vi "CMD_1.vi"(7 "JsonObj_Ori":refnum<class "JSON Value.lvclass">, 8 "error in (no error)":errorcluster, 9 "F/T":cluster{"Rack":string, "DUT Status":string[]}[](array[cluster])=[{"Rack"="201", "DUT Status"=["READY", "READY", "MAINTAIN", "CLOSE", "TEST"]}, {"Rack"="202", "DUT Status"=["READY", "READY", "MAINTAIN", "READY", "READY"]}], 10 "F/T-B":cluster{"Rack":string, "DUT Status":string[]}[](array[cluster])=[{"Rack"="101", "DUT Status"=["READY", "READY", "MAINTAIN", "CLOSE", "TEST"]}, {"Rack"="102", "DUT Status"=["READY", "READY", "MAINTAIN", "READY", "READY"]}], 11 "H/P":cluster{"Rack":string, "DUT Status":string[]}[](array[cluster])=[{"Rack"="1", "DUT Status"=[]}]) -> (0 "error out":errorcluster, 3 "Result":T1)   [LabVIEW 2020]
uses:
  <vilib>/addons/JSON API/JSON Value/JSON Value.lvclass
  <vilib>/addons/JSON API/JSON Value/Set from JSON string.vi
  <vilib>/addons/JSON API/JSON Value/Set sub-Item by names.vi
  <vilib>/addons/JSON API/JSON Scalar/JSON Scalar.lvclass
  C:/Program Files/National Instruments/LabVIEW 2020/vi.lib/addons/JSON API/JSON Value/JSON Value.lvclass
  <vilib>/addons/JSON API/JSON Array/JSON Array.lvclass
  <vilib>/addons/JSON API/JSON Value/Get sub-Item by names.vi
  <vilib>/addons/JSON API/JSON Scalar/Set String.vi
  <vilib>/addons/JSON API/JSON Value/Set Item by name array.vi
  <vilib>/addons/JSON API/JSON Array/Set JSON Array.vi
  <vilib>/addons/JSON API/JSON Value/Get as JSON string (pretty).vi
  <vilib>/addons/JSON API/Get Polymorphic/JSON GetSet.lvlib
  C:/Program Files/National Instruments/LabVIEW 2020/vi.lib/addons/JSON API/JSON Scalar/JSON Scalar.lvclass
  C:/Program Files/National Instruments/LabVIEW 2020/vi.lib/addons/JSON API/JSON Array/JSON Array.lvclass
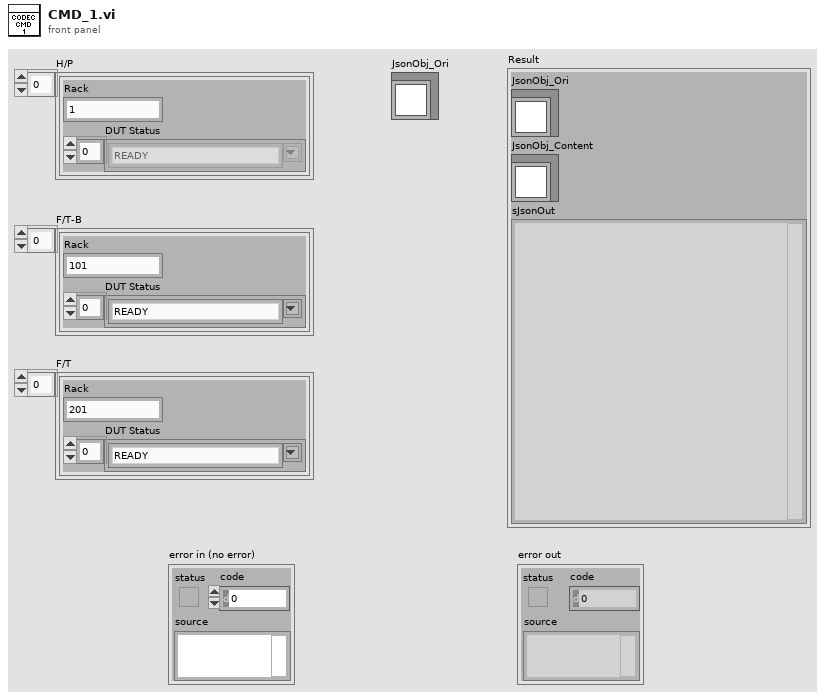
[diagram p1: front panel]
types:
  T1 = cluster{"JsonObj_Ori":refnum<class "JSON Value.lvclass">, "JsonObj_Content":refnum<class "JSON Value.lvclass">, "sJsonOut":string}
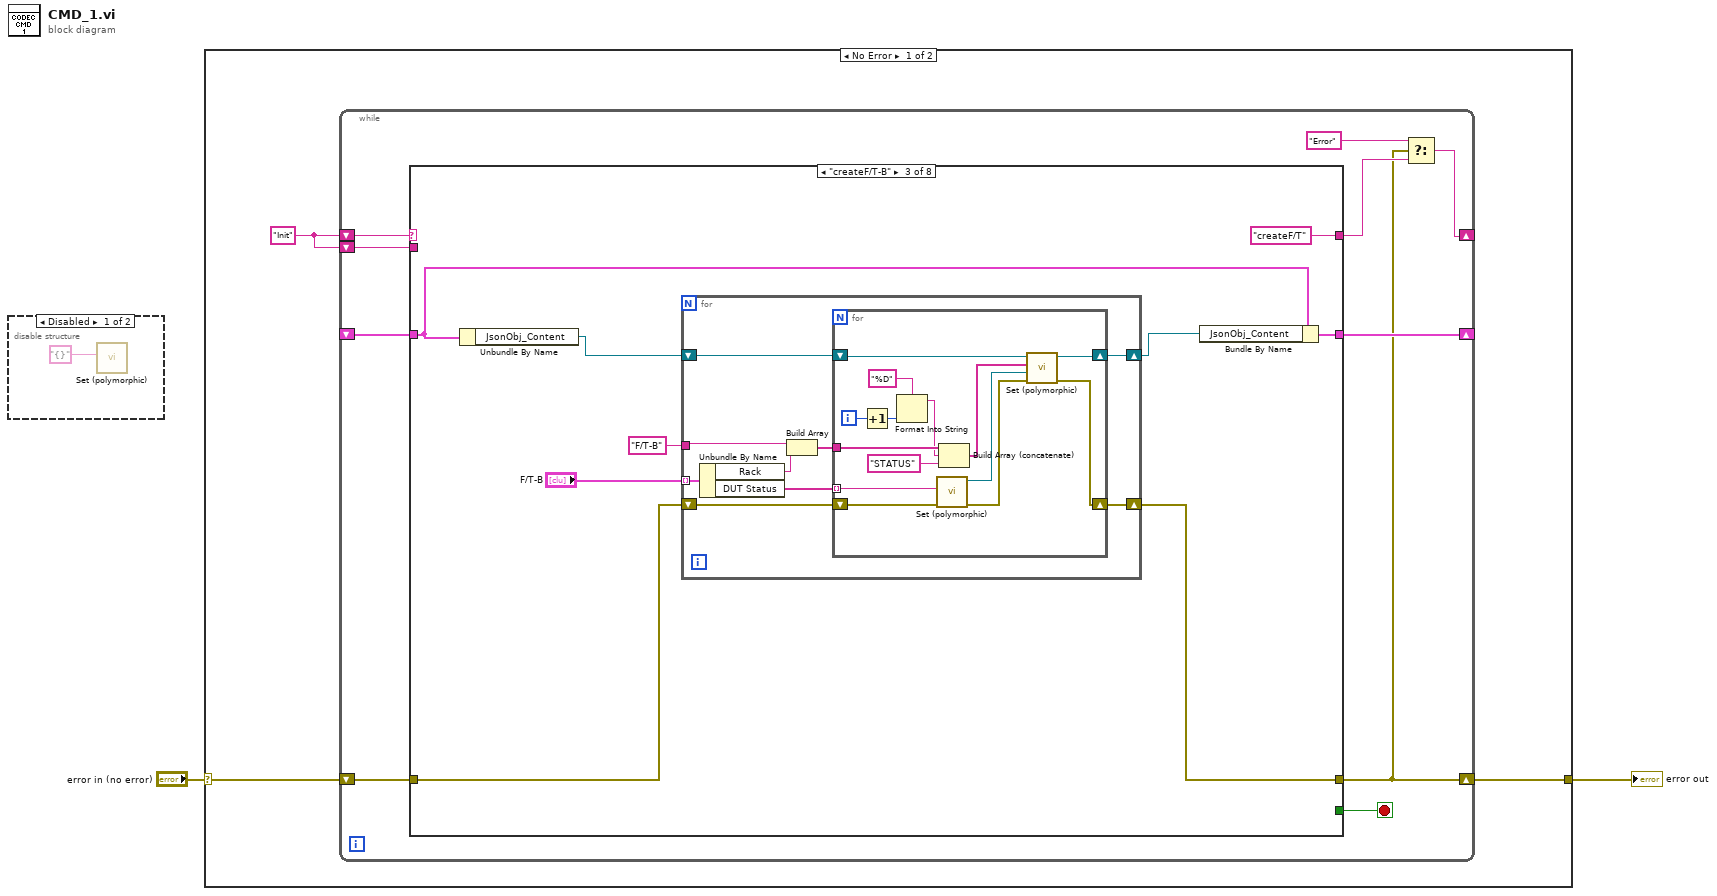
[diagram p0: block diagram]
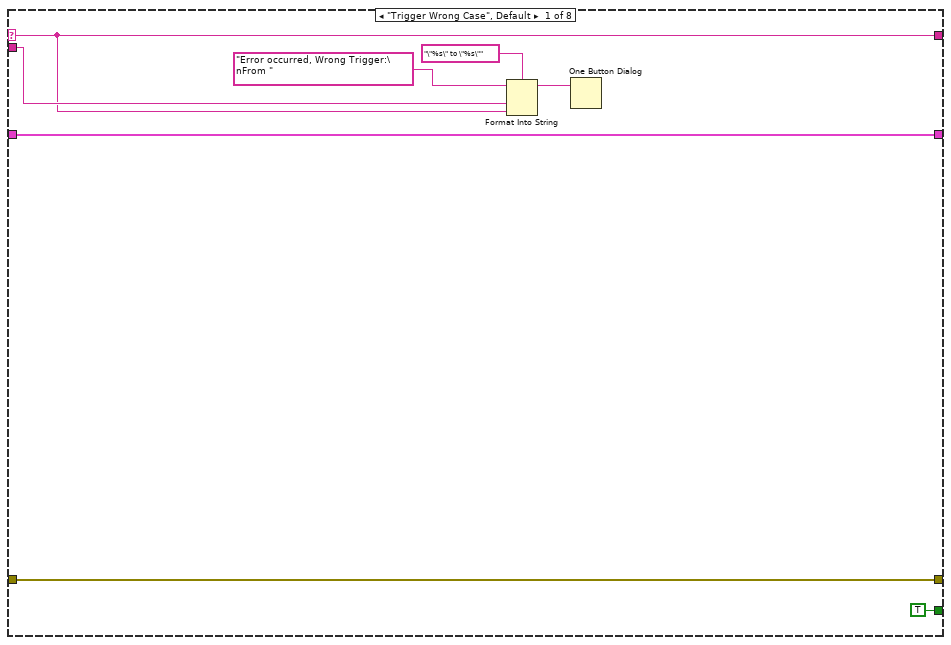
[diagram p3: hidden frame]
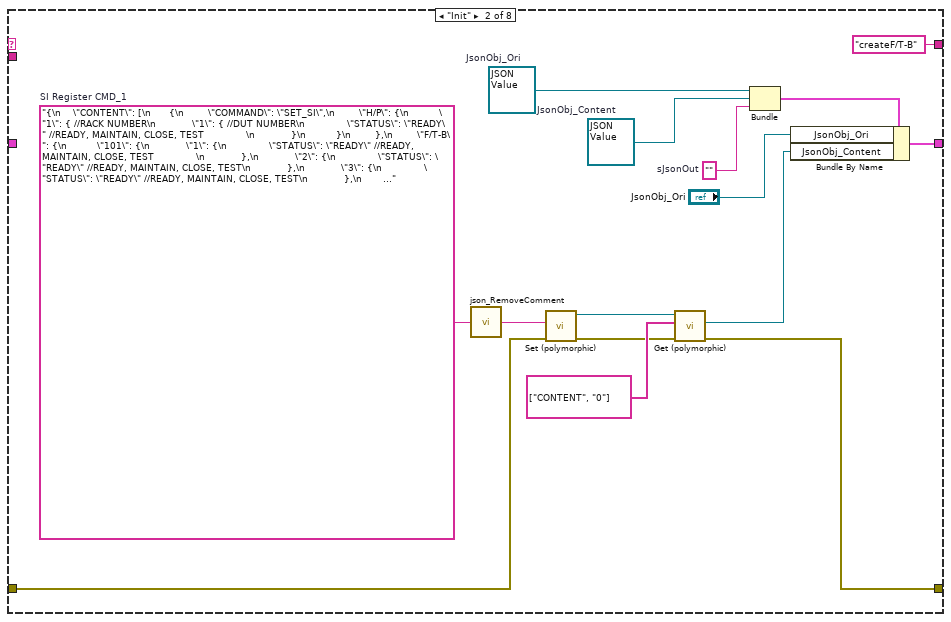
[diagram p4: hidden frame]
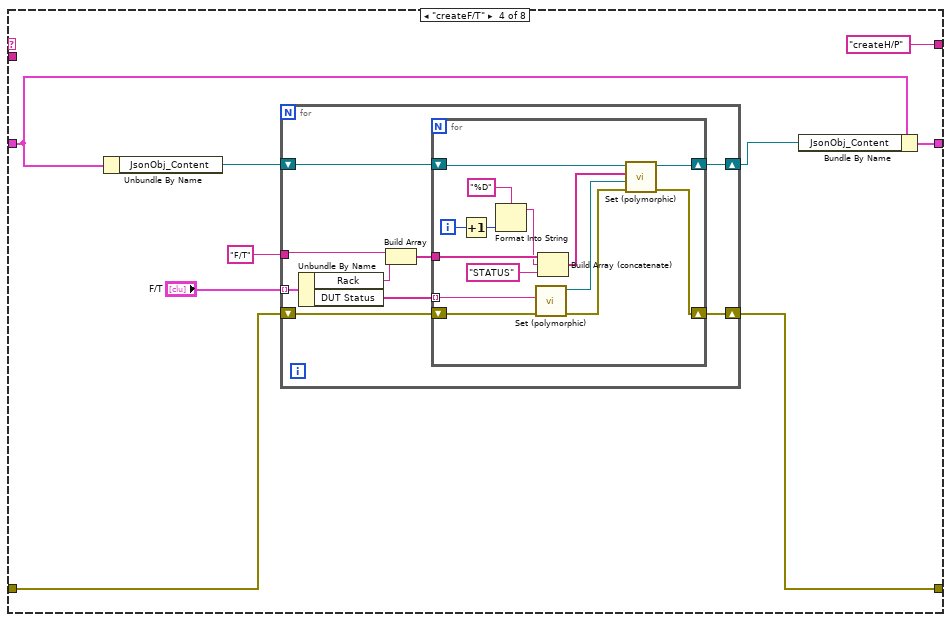
[diagram p5: hidden frame]
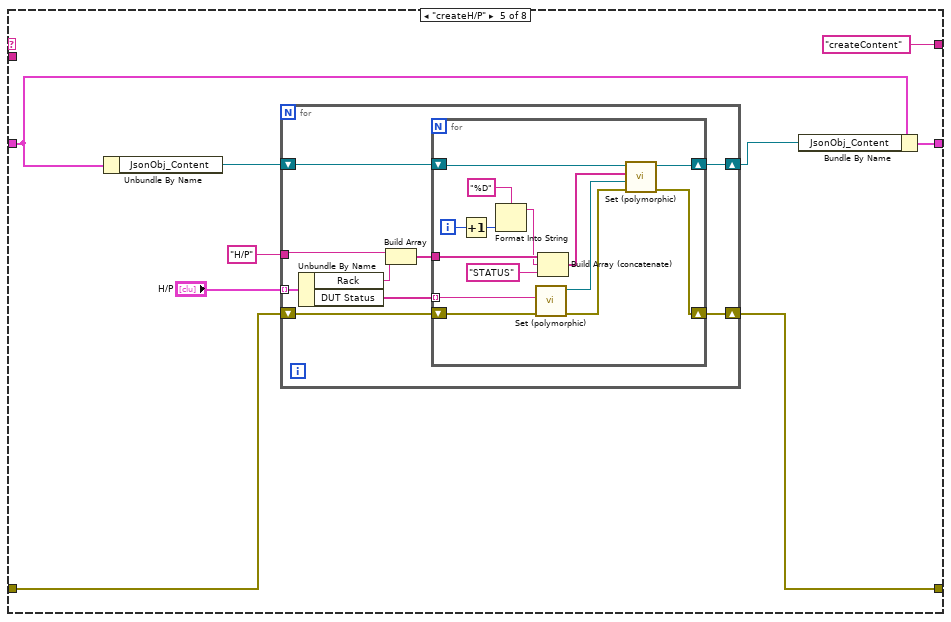
[diagram p6: hidden frame]
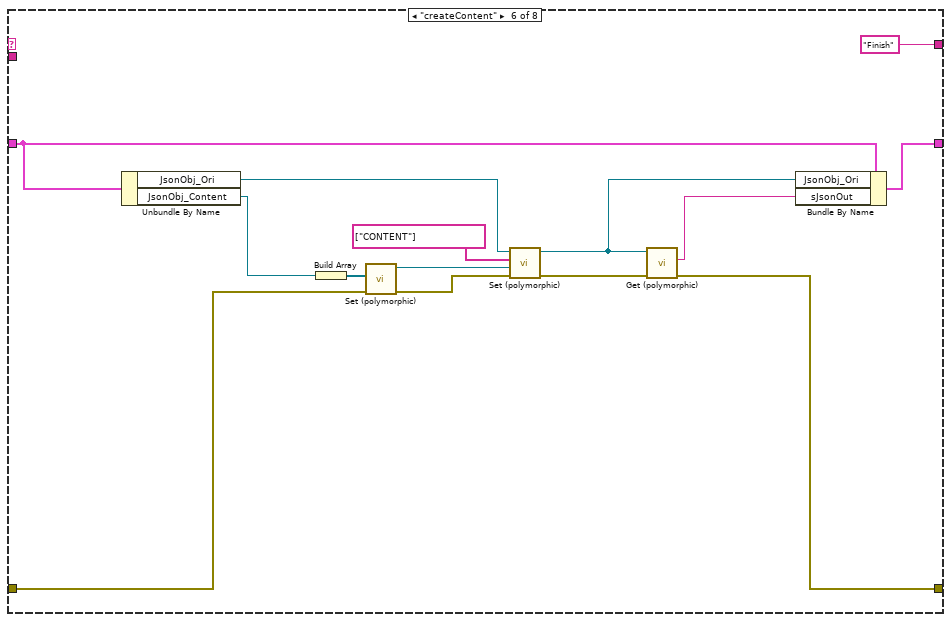
[diagram p7: hidden frame]
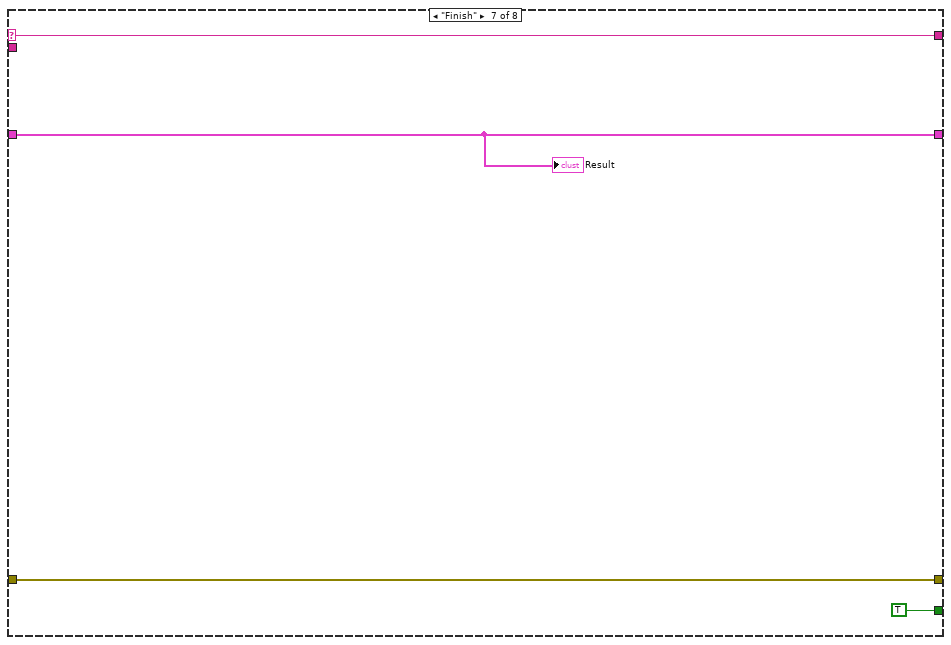
[diagram p8: hidden frame]
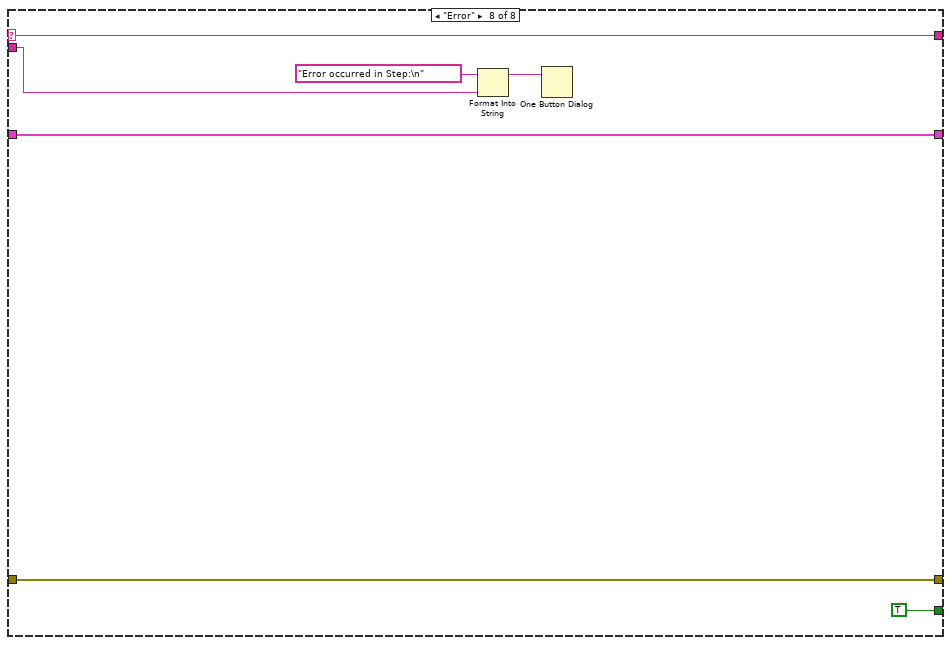
[diagram p9: hidden frame]
diagram:
  n1 = disable-structure shown="Disabled" {
    frame Disabled {
      n2 = call-poly <vilib>:"Set (polymorphic).vi"("JSON stream"="{}" ("JSON")) -> ()  [unwired: 8 in, 3 out]
    }
    frame Enabled {
    }
  }
  n3 = case shown="No Error" "error in (no error)" {
    selector: "error in (no error)" -> [w5 w161]
    tunnel: [w4 w161] -> w2
    frame No Error {
      w6 = "Init"
      n4 = while {
        shift-right: [w12] -> _
        shift-left: w6 -> [w16]
        shift-left: w6 -> [w15]
        shift-right: [w8] -> w4
        shift-left: w5 -> [w11]
        shift-right: [w10] -> _
        shift-left: _ -> [w9]
        stop <- w7 stop-if-true
        n5 = case shown="\"createF/T-B\"" w16 {
          selector: w16 -> [w20 _ _ _ _ _ w153 w160]
          tunnel: w15 -> [w21 _ _ _ _ _ _ w154]
          tunnel: [w20 "createF/T-B" "createF/T" "createH/P" "createContent" "Finish" w153 w160] -> w13
          tunnel: w11 -> [w19 w35 w44 w76 w108 w144 w151 w158]
          tunnel: [w19 w26 w43 w75 w107 w137 w151 w158] -> w8
          tunnel: [w18 w34 w48 w80 w112 w141 w152 w159] -> w10
          tunnel: w9 -> [w18 _ w41 w73 w105 w142 w152 w159]
          tunnel: [TRUE _ _ _ _ _ TRUE TRUE] -> w7
          frame "Trigger Wrong Case", Default {
            n6 = Format Into String(format string="\"%s\" to \"%s\"", initial string="Error occurred, Wrong Trigger:\nFrom ", w21, w20) -> (resulting string=w24:string)  [unwired: 1 in, 1 out]
            n7 = One Button Dialog(message=w24) -> ()  [unwired: 1 in, 1 out]
          }
          frame "Init" {
            w31 = ""  # sJsonOut
            w32 = refnum<class "JSON Value.lvclass"> refnum  # JsonObj_Content
            w37 = refnum<class "JSON Value.lvclass"> refnum  # JsonObj_Ori
            w39 = "{\n    \"CONTENT\": [\n      {\n        \"COMMAND\": \"SET_SI\",\n        \"H/P\": {\n          \"1\": { //RACK NUMBER\n            \"1\": { //DUT NUMBER\n              \"STATUS\": \"READY\" //READY, MAINTAIN, CLOSE, TEST              \n            }\n          }\n        },\n        \"F/T-B\": {\n          \"101\": {\n            \"1\": {\n              \"STATUS\": \"READY\" //READY, MAINTAIN, CLOSE, TEST              \n            },\n            \"2\": {\n              \"STATUS\": \"READY\" //READY, MAINTAIN, CLOSE, TEST\n            },\n            \"3\": {\n              \"STATUS\": \"READY\" //READY, MAINTAIN, CLOSE, TEST\n            },\n            \"4\": {\n              \"STATUS\": \"READY\" //READY, MAINTAIN, CLOSE, TEST\n            },\n            \"5\": {\n              \"STATUS\": \"READY\" //READY, MAINTAIN, CLOSE, TEST\n            }\n          },\n          \"102\": {\n            \"1\": {\n              \"STATUS\": \"READY\" //READY, MAINTAIN, CLOSE, TEST              \n            },\n            \"2\": {\n              \"STATUS\": \"READY\" //READY, MAINTAIN, CLOSE, TEST\n            },\n            \"3\": {\n              \"STATUS\": \"READY\" //READY, MAINTAIN, CLOSE, TEST\n            },\n            \"4\": {\n              \"STATUS\": \"READY\" //READY, MAINTAIN, CLOSE, TEST\n            },\n            \"5\": {\n              \"STATUS\": \"READY\" //READY, MAINTAIN, CLOSE, TEST\n            }\n          },\n          \"103\": {\n            \"1\": {\n              \"STATUS\": \"READY\" //READY, MAINTAIN, CLOSE, TEST              \n            },\n            \"2\": {\n              \"STATUS\": \"READY\" //READY, MAINTAIN, CLOSE, TEST\n            },\n            \"3\": {\n              \"STATUS\": \"READY\" //READY, MAINTAIN, CLOSE, TEST\n            },\n            \"4\": {\n              \"STATUS\": \"READY\" //READY, MAINTAIN, CLOSE, TEST\n            },\n            \"5\": {\n              \"STATUS\": \"READY\" //READY, MAINTAIN, CLOSE, TEST\n            }\n          },\n          \"104\": {\n            \"1\": {\n              \"STATUS\": \"READY\" //READY, MAINTAIN, CLOSE, TEST              \n            },\n            \"2\": {\n              \"STATUS\": \"READY\" //READY, MAINTAIN, CLOSE, TEST\n            },\n            \"3\": {\n              \"STATUS\": \"READY\" //READY, MAINTAIN, CLOSE, TEST\n            },\n            \"4\": {\n              \"STATUS\": \"READY\" //READY, MAINTAIN, CLOSE, TEST\n            },\n            \"5\": {\n              \"STATUS\": \"READY\" //READY, MAINTAIN, CLOSE, TEST\n            }\n          },\n          \"105\": {\n            \"1\": {\n              \"STATUS\": \"READY\" //READY, MAINTAIN, CLOSE, TEST              \n            },\n            \"2\": {\n              \"STATUS\": \"READY\" //READY, MAINTAIN, CLOSE, TEST\n            },\n            \"3\": {\n              \"STATUS\": \"READY\" //READY, MAINTAIN, CLOSE, TEST\n            },\n            \"4\": {\n              \"STATUS\": \"READY\" //READY, MAINTAIN, CLOSE, TEST\n            },\n            \"5\": {\n              \"STATUS\": \"READY\" //READY, MAINTAIN, CLOSE, TEST\n            }\n          },\n          \"106\": {\n            \"1\": {\n              \"STATUS\": \"READY\" //READY, MAINTAIN, CLOSE, TEST              \n            },\n            \"2\": {\n              \"STATUS\": \"READY\" //READY, MAINTAIN, CLOSE, TEST\n            },\n            \"3\": {\n              \"STATUS\": \"READY\" //READY, MAINTAIN, CLOSE, TEST\n            },\n            \"4\": {\n              \"STATUS\": \"READY\" //READY, MAINTAIN, CLOSE, TEST\n            },\n            \"5\": {\n              \"STATUS\": \"READY\" //READY, MAINTAIN, CLOSE, TEST\n            }\n          },\n          \"107\": {\n            \"1\": {\n              \"STATUS\": \"READY\" //READY, MAINTAIN, CLOSE, TEST              \n            },\n            \"2\": {\n              \"STATUS\": \"READY\" //READY, MAINTAIN, CLOSE, TEST\n            },\n            \"3\": {\n              \"STATUS\": \"READY\" //READY, MAINTAIN, CLOSE, TEST\n            },\n            \"4\": {\n              \"STATUS\": \"READY\" //READY, MAINTAIN, CLOSE, TEST\n            },\n            \"5\": {\n              \"STATUS\": \"READY\" //READY, MAINTAIN, CLOSE, TEST\n            }\n          },\n          \"108\": {\n            \"1\": {\n              \"STATUS\": \"READY\" //READY, MAINTAIN, CLOSE, TEST              \n            },\n            \"2\": {\n              \"STATUS\": \"READY\" //READY, MAINTAIN, CLOSE, TEST\n            },\n            \"3\": {\n              \"STATUS\": \"READY\" //READY, MAINTAIN, CLOSE, TEST\n            },\n            \"4\": {\n              \"STATUS\": \"READY\" //READY, MAINTAIN, CLOSE, TEST\n            },\n            \"5\": {\n              \"STATUS\": \"READY\" //READY, MAINTAIN, CLOSE, TEST\n            }\n          },\n          \"109\": {\n            \"1\": {\n              \"STATUS\": \"READY\" //READY, MAINTAIN, CLOSE, TEST              \n            },\n            \"2\": {\n              \"STATUS\": \"READY\" //READY, MAINTAIN, CLOSE, TEST\n            },\n            \"3\": {\n              \"STATUS\": \"READY\" //READY, MAINTAIN, CLOSE, TEST\n            },\n            \"4\": {\n              \"STATUS\": \"READY\" //READY, MAINTAIN, CLOSE, TEST\n            },\n            \"5\": {\n              \"STATUS\": \"READY\" //READY, MAINTAIN, CLOSE, TEST\n            }\n          },\n          \"110\": {\n            \"1\": {\n              \"STATUS\": \"READY\" //READY, MAINTAIN, CLOSE, TEST              \n            },\n            \"2\": {\n              \"STATUS\": \"READY\" //READY, MAINTAIN, CLOSE, TEST\n            },\n            \"3\": {\n              \"STATUS\": \"READY\" //READY, MAINTAIN, CLOSE, TEST\n            },\n            \"4\": {\n              \"STATUS\": \"READY\" //READY, MAINTAIN, CLOSE, TEST\n            },\n            \"5\": {\n              \"STATUS\": \"READY\" //READY, MAINTAIN, CLOSE, TEST\n            }\n          },\n          \"111\": {\n            \"1\": {\n              \"STATUS\": \"READY\" //READY, MAINTAIN, CLOSE, TEST              \n            },\n            \"2\": {\n              \"STATUS\": \"READY\" //READY, MAINTAIN, CLOSE, TEST\n            },\n            \"3\": {\n              \"STATUS\": \"READY\" //READY, MAINTAIN, CLOSE, TEST\n            },\n            \"4\": {\n              \"STATUS\": \"READY\" //READY, MAINTAIN, CLOSE, TEST\n            },\n            \"5\": {\n              \"STATUS\": \"READY\" //READY, MAINTAIN, CLOSE, TEST\n            }\n          },\n          \"112\": {\n            \"1\": {\n              \"STATUS\": \"READY\" //READY, MAINTAIN, CLOSE, TEST              \n            },\n            \"2\": {\n              \"STATUS\": \"READY\" //READY, MAINTAIN, CLOSE, TEST\n            },\n            \"3\": {\n              \"STATUS\": \"READY\" //READY, MAINTAIN, CLOSE, TEST\n            },\n            \"4\": {\n              \"STATUS\": \"READY\" //READY, MAINTAIN, CLOSE, TEST\n            },\n            \"5\": {\n              \"STATUS\": \"READY\" //READY, MAINTAIN, CLOSE, TEST\n            }\n          }\n        },\n        \"F/T\": {\n          \"201\": {\n            \"1\": {\n              \"STATUS\": \"READY\" //READY, MAINTAIN, CLOSE, TEST              \n            },\n            \"2\": {\n              \"STATUS\": \"READY\" //READY, MAINTAIN, CLOSE, TEST\n            },\n            \"3\": {\n              \"STATUS\": \"READY\" //READY, MAINTAIN, CLOSE, TEST\n            },\n            \"4\": {\n              \"STATUS\": \"READY\" //READY, MAINTAIN, CLOSE, TEST\n            },\n            \"5\": {\n              \"STATUS\": \"READY\" //READY, MAINTAIN, CLOSE, TEST\n            }\n          },\n          \"202\": {\n            \"1\": {\n              \"STATUS\": \"READY\" //READY, MAINTAIN, CLOSE, TEST              \n            },\n            \"2\": {\n              \"STATUS\": \"READY\" //READY, MAINTAIN, CLOSE, TEST\n            },\n            \"3\": {\n              \"STATUS\": \"READY\" //READY, MAINTAIN, CLOSE, TEST\n            },\n            \"4\": {\n              \"STATUS\": \"READY\" //READY, MAINTAIN, CLOSE, TEST\n            },\n            \"5\": {\n              \"STATUS\": \"READY\" //READY, MAINTAIN, CLOSE, TEST\n            }\n          },\n          \"203\": {\n            \"1\": {\n              \"STATUS\": \"READY\" //READY, MAINTAIN, CLOSE, TEST              \n            },\n            \"2\": {\n              \"STATUS\": \"READY\" //READY, MAINTAIN, CLOSE, TEST\n            },\n            \"3\": {\n              \"STATUS\": \"READY\" //READY, MAINTAIN, CLOSE, TEST\n            },\n            \"4\": {\n              \"STATUS\": \"READY\" //READY, MAINTAIN, CLOSE, TEST\n            },\n            \"5\": {\n              \"STATUS\": \"READY\" //READY, MAINTAIN, CLOSE, TEST\n            }\n          },\n          \"204\": {\n            \"1\": {\n              \"STATUS\": \"READY\" //READY, MAINTAIN, CLOSE, TEST              \n            },\n            \"2\": {\n              \"STATUS\": \"READY\" //READY, MAINTAIN, CLOSE, TEST\n            },\n            \"3\": {\n              \"STATUS\": \"READY\" //READY, MAINTAIN, CLOSE, TEST\n            },\n            \"4\": {\n              \"STATUS\": \"READY\" //READY, MAINTAIN, CLOSE, TEST\n            },\n            \"5\": {\n              \"STATUS\": \"READY\" //READY, MAINTAIN, CLOSE, TEST\n            }\n          },\n          \"205\": {\n            \"1\": {\n              \"STATUS\": \"READY\" //READY, MAINTAIN, CLOSE, TEST              \n            },\n            \"2\": {\n              \"STATUS\": \"READY\" //READY, MAINTAIN, CLOSE, TEST\n            },\n            \"3\": {\n              \"STATUS\": \"READY\" //READY, MAINTAIN, CLOSE, TEST\n            },\n            \"4\": {\n              \"STATUS\": \"READY\" //READY, MAINTAIN, CLOSE, TEST\n            },\n            \"5\": {\n              \"STATUS\": \"READY\" //READY, MAINTAIN, CLOSE, TEST\n            }\n          },\n          \"206\": {\n            \"1\": {\n              \"STATUS\": \"READY\" //READY, MAINTAIN, CLOSE, TEST              \n            },\n            \"2\": {\n              \"STATUS\": \"READY\" //READY, MAINTAIN, CLOSE, TEST\n            },\n            \"3\": {\n              \"STATUS\": \"READY\" //READY, MAINTAIN, CLOSE, TEST\n            },\n            \"4\": {\n              \"STATUS\": \"READY\" //READY, MAINTAIN, CLOSE, TEST\n            },\n            \"5\": {\n              \"STATUS\": \"READY\" //READY, MAINTAIN, CLOSE, TEST\n            }\n          },\n          \"207\": {\n            \"1\": {\n              \"STATUS\": \"READY\" //READY, MAINTAIN, CLOSE, TEST              \n            },\n            \"2\": {\n              \"STATUS\": \"READY\" //READY, MAINTAIN, CLOSE, TEST\n            },\n            \"3\": {\n              \"STATUS\": \"READY\" //READY, MAINTAIN, CLOSE, TEST\n            },\n            \"4\": {\n              \"STATUS\": \"READY\" //READY, MAINTAIN, CLOSE, TEST\n            },\n            \"5\": {\n              \"STATUS\": \"READY\" //READY, MAINTAIN, CLOSE, TEST\n            }\n          },\n          \"208\": {\n            \"1\": {\n              \"STATUS\": \"READY\" //READY, MAINTAIN, CLOSE, TEST              \n            },\n            \"2\": {\n              \"STATUS\": \"READY\" //READY, MAINTAIN, CLOSE, TEST\n            },\n            \"3\": {\n              \"STATUS\": \"READY\" //READY, MAINTAIN, CLOSE, TEST\n            },\n            \"4\": {\n              \"STATUS\": \"READY\" //READY, MAINTAIN, CLOSE, TEST\n            },\n            \"5\": {\n              \"STATUS\": \"READY\" //READY, MAINTAIN, CLOSE, TEST\n            }\n          },\n          \"209\": {\n            \"1\": {\n              \"STATUS\": \"READY\" //READY, MAINTAIN, CLOSE, TEST              \n            },\n            \"2\": {\n              \"STATUS\": \"READY\" //READY, MAINTAIN, CLOSE, TEST\n            },\n            \"3\": {\n              \"STATUS\": \"READY\" //READY, MAINTAIN, CLOSE, TEST\n            },\n            \"4\": {\n              \"STATUS\": \"READY\" //READY, MAINTAIN, CLOSE, TEST\n            },\n            \"5\": {\n              \"STATUS\": \"READY\" //READY, MAINTAIN, CLOSE, TEST\n            }\n          },\n          \"210\": {\n            \"1\": {\n              \"STATUS\": \"READY\" //READY, MAINTAIN, CLOSE, TEST              \n            },\n            \"2\": {\n              \"STATUS\": \"READY\" //READY, MAINTAIN, CLOSE, TEST\n            },\n            \"3\": {\n              \"STATUS\": \"READY\" //READY, MAINTAIN, CLOSE, TEST\n            },\n            \"4\": {\n              \"STATUS\": \"READY\" //READY, MAINTAIN, CLOSE, TEST\n            },\n            \"5\": {\n              \"STATUS\": \"READY\" //READY, MAINTAIN, CLOSE, TEST\n            }\n          },\n          \"211\": {\n            \"1\": {\n              \"STATUS\": \"READY\" //READY, MAINTAIN, CLOSE, TEST              \n            },\n            \"2\": {\n              \"STATUS\": \"READY\" //READY, MAINTAIN, CLOSE, TEST\n            },\n            \"3\": {\n              \"STATUS\": \"READY\" //READY, MAINTAIN, CLOSE, TEST\n            },\n            \"4\": {\n              \"STATUS\": \"READY\" //READY, MAINTAIN, CLOSE, TEST\n            },\n            \"5\": {\n              \"STATUS\": \"READY\" //READY, MAINTAIN, CLOSE, TEST\n            }\n          },\n          \"212\": {\n            \"1\": {\n              \"STATUS\": \"READY\" //READY, MAINTAIN, CLOSE, TEST              \n            },\n            \"2\": {\n              \"STATUS\": \"READY\" //READY, MAINTAIN, CLOSE, TEST\n            },\n            \"3\": {\n              \"STATUS\": \"READY\" //READY, MAINTAIN, CLOSE, TEST\n            },\n            \"4\": {\n              \"STATUS\": \"READY\" //READY, MAINTAIN, CLOSE, TEST\n            },\n            \"5\": {\n              \"STATUS\": \"READY\" //READY, MAINTAIN, CLOSE, TEST\n            }\n          }\n        }\n      }\n    ]\n  }"  # SI Register CMD_1
            n8 = call "json_RemoveComment.vi"("json with comment"=w39) -> ("json without comment"=w38:string)
            n9 = call-poly <vilib>:"Set (polymorphic).vi"("error in (no error)"=w35, "JSON stream"=w38) -> ("error out"=w27:errorcluster, "JSON Value out"=w30:refnum<class "JSON Value.lvclass">)  [unwired: 7 in, 1 out]
            n10 = call-poly <vilib>:"Get (polymorphic).vi"("error in (no error)"=w27, "Name Array"=string[] ["CONTENT", "0"], "JSON Value In"=w30) -> ("error out"=w26:errorcluster, "Value"=w28:refnum<class "JSON Value.lvclass">)  [unwired: 5 in, 2 out]
            n11 = Bundle("JsonObj_Ori"=w37, "JsonObj_Content"=w32, "sJsonOut"=w31) -> (w36:T1)  [unwired: 1 in]
            n12 = Bundle By Name(cluster=w36, "JsonObj_Ori"="JsonObj_Ori", "JsonObj_Content"=w28) -> (w34:T1)
          }
          frame "createF/T-B" {
            n13 = Unbundle By Name(w41) -> ("JsonObj_Content"=w40:refnum<class "JSON Value.lvclass">)
            n14 = for {
              tunnel: "F/T-B" -> [w57] mode=indexing
              tunnel: "F/T-B" ("name") -> [w56]
              shift-right: [w52] -> w42
              shift-left: w40 -> [w53]
              shift-right: [w49] -> w43
              shift-left: w44 -> [w50]
              n15 = Unbundle By Name(w57) -> ("Rack"=w55:string, "DUT Status"=w54:string[])
              n16 = Build Array(w56, w55) -> (w51:string[])
              n17 = for {
                tunnel: w54 -> [w71] mode=indexing
                shift-right: [w69] -> w52
                shift-left: w53 -> [w70]
                tunnel: w51 -> [w64]
                shift-right: [w58] -> w49
                shift-left: w50 -> [w60]
                i -> [w65]
                n18 = Increment(x=w65) -> (x+1=w67:i32)
                n19 = Format Into String(format string="%D", w67) -> (resulting string=w63:string)  [unwired: 2 in, 1 out]
                n20 = call-poly <vilib>:"Set (polymorphic).vi"("error in (no error)"=w60, "String"=w71) -> ("error out"=w59:errorcluster, "JSON Scalar out"=w68:refnum<class "JSON Scalar.lvclass">)  [unwired: 8 in]
                n21 = Build Array (concatenate)(w64, w63, "STATUS" ("element")) -> (w62:string[])
                n22 = call-poly <vilib>:"Set (polymorphic).vi"("error in (no error)"=w59, "Value"=w68, "Name Array"=w62, "JSON Value In"=w70) -> ("error out"=w58:errorcluster, "JSON Value Out"=w69:refnum<class "JSON Value.lvclass">)  [unwired: 5 in, 1 out]
              }
            }
            n23 = Bundle By Name(cluster=w41, "JsonObj_Content"=w42) -> (w48:T1)
          }
          frame "createF/T" {
            n24 = Unbundle By Name(w73) -> ("JsonObj_Content"=w72:refnum<class "JSON Value.lvclass">)
            n25 = for {
              tunnel: "F/T" -> [w89] mode=indexing
              tunnel: "F/T" ("name") -> [w88]
              shift-right: [w84] -> w74
              shift-left: w72 -> [w85]
              shift-right: [w81] -> w75
              shift-left: w76 -> [w82]
              n26 = Unbundle By Name(w89) -> ("Rack"=w87:string, "DUT Status"=w86:string[])
              n27 = Build Array(w88, w87) -> (w83:string[])
              n28 = for {
                tunnel: w86 -> [w103] mode=indexing
                shift-right: [w101] -> w84
                shift-left: w85 -> [w102]
                tunnel: w83 -> [w96]
                shift-right: [w90] -> w81
                shift-left: w82 -> [w92]
                i -> [w97]
                n29 = Increment(x=w97) -> (x+1=w99:i32)
                n30 = Format Into String(format string="%D", w99) -> (resulting string=w95:string)  [unwired: 2 in, 1 out]
                n31 = call-poly <vilib>:"Set (polymorphic).vi"("error in (no error)"=w92, "String"=w103) -> ("error out"=w91:errorcluster, "JSON Scalar out"=w100:refnum<class "JSON Scalar.lvclass">)  [unwired: 8 in]
                n32 = Build Array (concatenate)(w96, w95, "STATUS" ("element")) -> (w94:string[])
                n33 = call-poly <vilib>:"Set (polymorphic).vi"("error in (no error)"=w91, "Value"=w100, "Name Array"=w94, "JSON Value In"=w102) -> ("error out"=w90:errorcluster, "JSON Value Out"=w101:refnum<class "JSON Value.lvclass">)  [unwired: 5 in, 1 out]
              }
            }
            n34 = Bundle By Name(cluster=w73, "JsonObj_Content"=w74) -> (w80:T1)
          }
          frame "createH/P" {
            n35 = Unbundle By Name(w105) -> ("JsonObj_Content"=w104:refnum<class "JSON Value.lvclass">)
            n36 = for {
              tunnel: "H/P" -> [w121] mode=indexing
              tunnel: "H/P" ("name") -> [w120]
              shift-right: [w116] -> w106
              shift-left: w104 -> [w117]
              shift-right: [w113] -> w107
              shift-left: w108 -> [w114]
              n37 = Unbundle By Name(w121) -> ("Rack"=w119:string, "DUT Status"=w118:string[])
              n38 = Build Array(w120, w119) -> (w115:string[])
              n39 = for {
                tunnel: w118 -> [w135] mode=indexing
                shift-right: [w133] -> w116
                shift-left: w117 -> [w134]
                tunnel: w115 -> [w128]
                shift-right: [w122] -> w113
                shift-left: w114 -> [w124]
                i -> [w129]
                n40 = Increment(x=w129) -> (x+1=w131:i32)
                n41 = Format Into String(format string="%D", w131) -> (resulting string=w127:string)  [unwired: 2 in, 1 out]
                n42 = call-poly <vilib>:"Set (polymorphic).vi"("error in (no error)"=w124, "String"=w135) -> ("error out"=w123:errorcluster, "JSON Scalar out"=w132:refnum<class "JSON Scalar.lvclass">)  [unwired: 8 in]
                n43 = Build Array (concatenate)(w128, w127, "STATUS" ("element")) -> (w126:string[])
                n44 = call-poly <vilib>:"Set (polymorphic).vi"("error in (no error)"=w123, "Value"=w132, "Name Array"=w126, "JSON Value In"=w134) -> ("error out"=w122:errorcluster, "JSON Value Out"=w133:refnum<class "JSON Value.lvclass">)  [unwired: 5 in, 1 out]
              }
            }
            n45 = Bundle By Name(cluster=w105, "JsonObj_Content"=w106) -> (w112:T1)
          }
          frame "createContent" {
            n46 = Unbundle By Name(w142) -> ("JsonObj_Ori"=w145:refnum<class "JSON Value.lvclass">, "JsonObj_Content"=w146:refnum<class "JSON Value.lvclass">)
            n47 = Build Array(w146) -> (w147:refnum<class "JSON Value.lvclass">[])
            n48 = call-poly <vilib>:"Set (polymorphic).vi"("error in (no error)"=w144, "Array"=w147) -> ("error out"=w143:errorcluster, "JSON Array out"=w148:refnum<class "JSON Array.lvclass">)  [unwired: 8 in]
            n49 = call-poly <vilib>:"Set (polymorphic).vi"("error in (no error)"=w143, "Value"=w148, "Name Array"=string[] ["CONTENT"], "JSON Value In"=w145) -> ("error out"=w138:errorcluster, "JSON Value Out"=w140:refnum<class "JSON Value.lvclass">)  [unwired: 5 in, 1 out]
            n50 = call-poly <vilib>:"Get (polymorphic).vi"("error in (no error)"=w138, "JSON Value in"=w140) -> ("error out"=w137:errorcluster, "<JSON>"=w139:string)  [unwired: 8 in]
            n51 = Bundle By Name(cluster=w142, "JsonObj_Ori"=w140, "sJsonOut"=w139) -> (w141:T1)
          }
          frame "Finish" {
            "Result" <- w152
          }
          frame "Error" {
            n52 = Format Into String(initial string="Error occurred in Step:\n", w154) -> (resulting string=w155:string)  [unwired: 2 in, 1 out]
            n53 = One Button Dialog(message=w155) -> ()  [unwired: 1 in, 1 out]
          }
        }
        n54 = Select(t="Error", s=w8, f=w13) -> (s? t:f=w12:string)
      }
    }
    frame Error {
    }
  }
  "error out" <- w2
